vi "Gear Ratio Correction.vi"(6 "PID gains input":T1={"proportional gain (Kc)"=0.01, "integral time (Ti, min)"=0.003, "derivative time (Td, min)"=0.0} {"derivative time (Td, min)" format="%.6f"; "integral time (Ti, min)" format="%.6f"; "proportional gain (Kc)" format="%.6f"}, 8 "error in":errorcluster, 9 "Motor in":dbl, 10 "Main motor's gear ratio":dbl=30.0, 11 "This motor's gear ratio":dbl=44.0) -> (0 "error out":errorcluster, 3 "Motor out":dbl, 4 "PID gains output":T1={"proportional gain (Kc)"=0.01, "integral time (Ti, min)"=0.003, "derivative time (Td, min)"=0.0} {"derivative time (Td, min)" format="%.6f"; "integral time (Ti, min)" format="%.6f"; "proportional gain (Kc)" format="%.6f"})   [LabVIEW 2016]
panel:
  # "VI Description: Adjust the output to a particular motor based on the ratio of the motor gearing."
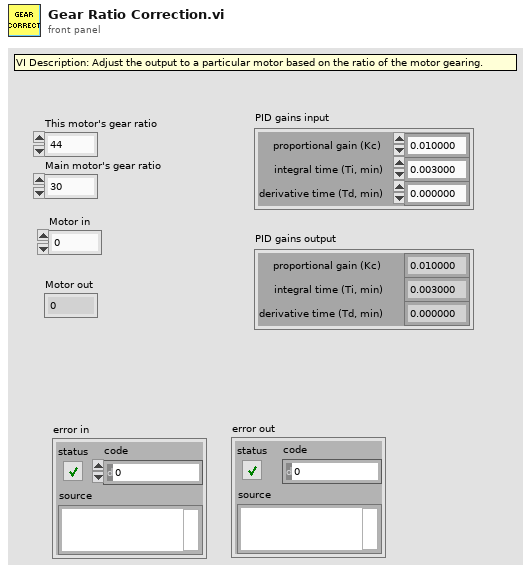
[diagram p1: front panel]
types:
  T1 = cluster{"proportional gain (Kc)":dbl, "integral time (Ti, min)":dbl, "derivative time (Td, min)":dbl}
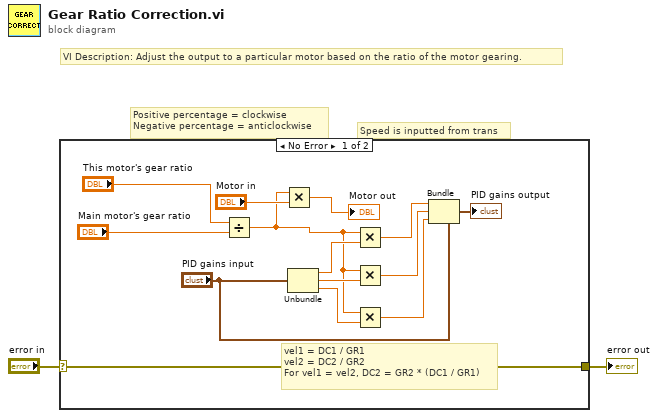
[diagram p0: block diagram]
diagram:
  # "VI Description: Adjust the output to a particular motor based on the ratio of the motor gearing."
  # "Positive percentage = clockwise\nNegative percentage = anticlockwise"
  # "Speed is inputted from trans"
  n1 = case shown="No Error" "error in" {
    selector: "error in" -> [w16 w17]
    tunnel: [w16 w17] -> w1
    frame No Error {
      # "vel1 = DC1 / GR1\nvel2 = DC2 / GR2\nFor vel1 = vel2, DC2 = GR2 * (DC1 / GR1)"
      n2 = Divide(x="This motor's gear ratio", y="Main motor's gear ratio") -> (x/y=w3:dbl)
      n3 = Multiply(x=w3, y="Motor in") -> (x*y=→"Motor out":dbl)
      n4 = Unbundle("PID gains input") -> ("proportional gain (Kc)"=w4:dbl, "integral time (Ti, min)"=w11:dbl, "derivative time (Td, min)"=w10:dbl)
      n5 = Multiply(x=w3, y=w4) -> (x*y=w8:dbl)
      n6 = Multiply(x=w3, y=w11) -> (x*y=w7:dbl)
      n7 = Multiply(x=w3, y=w10) -> (x*y=w6:dbl)
      n8 = Bundle(cluster="PID gains input", "proportional gain (Kc)"=w8, "integral time (Ti, min)"=w7, "derivative time (Td, min)"=w6) -> (→"PID gains output":T1)
    }
    frame Error {
    }
  }
  "error out" <- w1
